vi "Short Name to Path.vi"(8 "error in":errorcluster, 11 "LabVIEW Path":path) -> (0 "error out":errorcluster, 3 "UTF-8 Path":refnum<class "UTF-8 Path.lvclass">)   [LabVIEW 2020, in "G-Unicode.lvlib"]
doc: "Converts the LabVIEW path in 8.3 short name format to the corresponding unicode path. Note that the path must exist on disk.\n\n<b>Windows only.</b> Linux and macOS will return a UTF-8 encoded path."
uses:
  G-Unicode.lvlib
  f844562b-b612-4fa1-b092-3cf87b2107aa.vi
  kernel32.dll
  Types/UTF-8 Path/UTF-8 Path.lvclass
  Types/UTF-8 String/UTF-8 String.lvclass
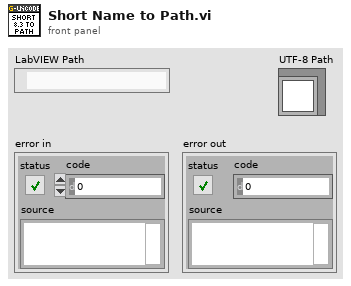
[diagram p1: front panel]
types:
  T1 = typedef "G-Unicode.lvlib/Encoded UTF-8 String.ctl" = string
  T2 = typedef "G-Unicode.lvlib/Encoded UTF-16LE String.ctl" = string
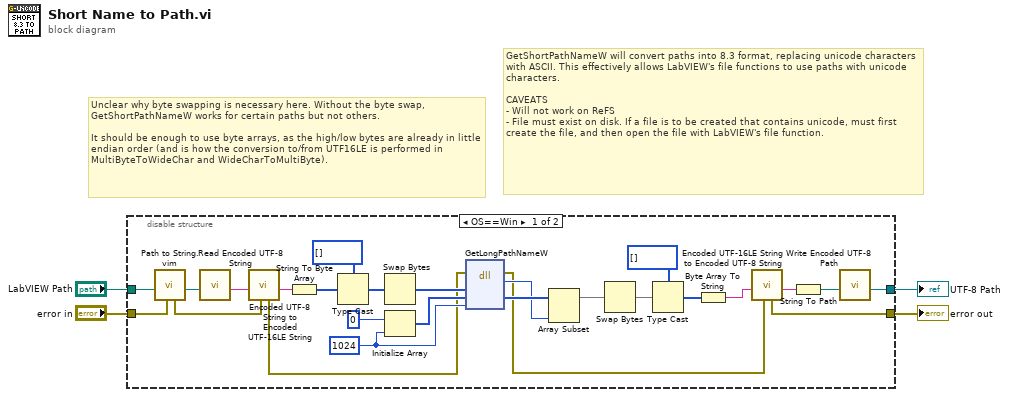
[diagram p0: block diagram]
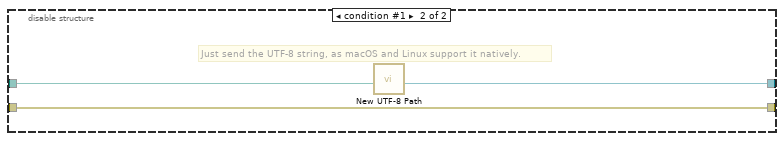
[diagram p2: hidden frame]
diagram:
  # "GetShortPathNameW will convert paths into 8.3 format, replacing unicode characters with ASCII. This effectively allows LabVIEW's file functions to use paths with unicode characters.\n\nCAVEATS\n- Will not work on ReFS\n- File must exist on disk. If a file is to be created that contains unicode, must first create the file, and then open the file with LabVIEW's file function."
  # "Unclear why byte swapping is necessary here. Without the byte swap, GetShortPathNameW works for certain paths but not others.\n\nIt should be enough to use byte arrays, as the high/low bytes are already in little endian order (and is how the conversion to/from UTF16LE is performed in MultiByteToWideChar and WideCharToMultiByte)."
  n1 = disable-structure shown="OS==Win" {
    disable-tunnel: [w10 w31] -> w1
    disable-tunnel: "LabVIEW Path" -> [w13 w32]
    disable-tunnel: "error in" -> [w12 w33]
    disable-tunnel: [w15 w33] -> w3
    frame condition #0 (active) {
      w28 = u32 1024 ("dimension size")
      n2 = call "Path to String.vim"("error in"=w12, "Path"=w13) -> ("String"=w7:refnum<class "UTF-8 String.lvclass">, "error out"=w5:errorcluster)  [unwired: 8 in]
      n3 = call "Read Encoded UTF-8 String.vi"("UTF-8 String"=w7) -> ("Encoded UTF-8 String"=w6:T1)  [unwired: 10 in]
      n4 = call "Encoded UTF-8 String to Encoded UTF-16LE String.vi"("error in"=w5, "Encoded UTF-8 String"=w6) -> ("Encoded UTF-16LE String"=w9:T2, "error out"=w8:errorcluster)  [unwired: 8 in]
      n5 = String To Byte Array(string=w9) -> (unsigned byte array=w21:u8[])
      n6 = Type Cast(type=u16[] [], x=w21) -> (*(type *) &x=w26:u16[])
      n7 = Swap Bytes(anything=w26) -> (byte swapped=w19:u16[])
      n8 = Initialize Array(u16 0 ("element"), w28) -> (w29:u16[])
      n9 = dll-call lib="kernel32.dll" fn="GetLongPathNameW"(error in=w8, "lpszShortPath"=w19, "lpszLongPath"=w29, "cchBuffer"=w28) -> (error out=w16:errorcluster, "return type"=w18:u32, "lpszLongPath"=w25:u16[])  [unwired: 4 in, 1 out]
      n10 = Array Subset(array=w25, length=w18) -> (w20:u16[])  [unwired: 1 in]
      n11 = Swap Bytes(anything=w20) -> (byte swapped=w23:u16[])
      n12 = Type Cast(type=u8[] [], x=w23) -> (*(type *) &x=w17:u8[])
      n13 = Byte Array To String(unsigned byte array=w17) -> (string=w27:string)
      n14 = call "Encoded UTF-16LE String to Encoded UTF-8 String.vi"("error in"=w16, "Encoded UTF-16LE String"=w27) -> ("Encoded UTF-8 String"=w14:T1, "error out"=w15:errorcluster)  [unwired: 8 in]
      n15 = String To Path(string=w14) -> (path=w11:path)
      n16 = call "Write Encoded UTF-8 Path.vi"("Encoded UTF-8 Path"=w11) -> ("UTF-8 Path"=w10:refnum<class "UTF-8 Path.lvclass">)  [unwired: 10 in]
    }
    frame condition #1 {
      # "Just send the UTF-8 string, as macOS and Linux support it natively."
      n17 = call "New UTF-8 Path.vi"("LabVIEW Path"=w32) -> ("UTF-8 Path"=w31:refnum<class "UTF-8 Path.lvclass">)  [unwired: 9 in, 1 out]
    }
  }
  "error out" <- w3
  "UTF-8 Path" <- w1
